vi "Write--move.vi"(8 "error in (no error)":errorcluster, 10 "Comando":T1 {"Tipo de paso" items=["Medio paso", "Paso completo"]; "Dirección" items=["Izquierda", "Derecha"]; "Tipo" items=["Unipolar", "Bipolar"]}, 11 "VISA resource name":refnum<visa-resource-name>) -> (0 "error out":errorcluster, 2 "Comando(string)":string, 3 "VISA resource name out":refnum<visa-resource-name>)   [LabVIEW 2020, in "Control de MaP.lvlib"]
doc: "Sends the move command to the MCU based in the parameters specified in the Command cluster. The MCU will be execute in a \"Moving\" state. You can send position, end-stop, all information and stop commands while in this state."
uses:
  Control de MaP.lvlib
  Controls/Command to motor.ctl
  <vilib>/Instr/_visa.llb/VISA Flush IO Buffer Mask.ctl
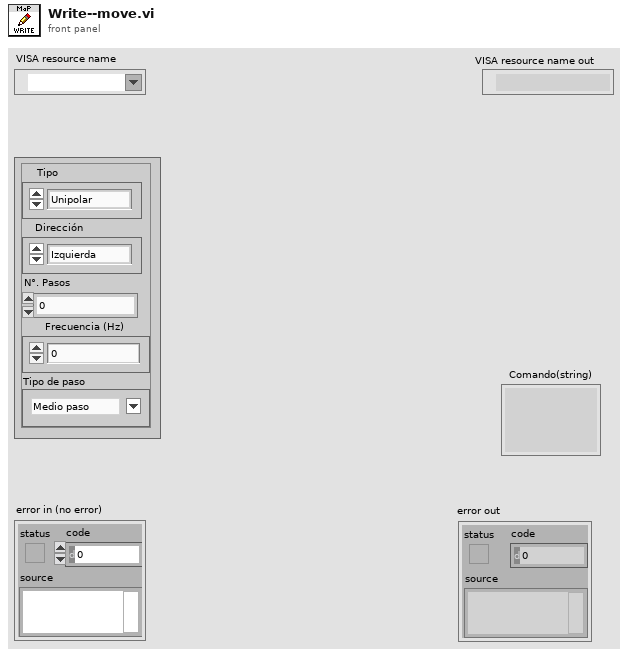
[diagram p1: front panel]
types:
  T1 = typedef "Control de MaP.lvlib/Command to motor.ctl" = cluster{"Tipo":u8, "Dirección":u8, "N°. Pasos":u16, "Frecuencia (Hz)":u8, "Tipo de paso":u8}
  T2 = typedef "VISA Flush IO Buffer Mask.ctl" = u16
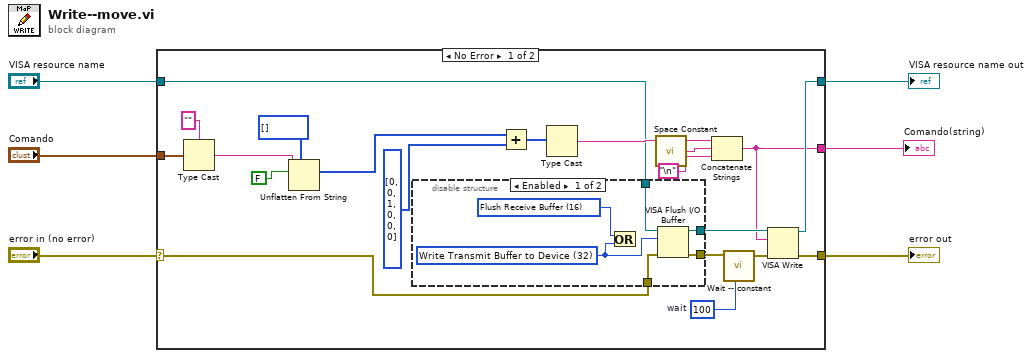
[diagram p0: block diagram]
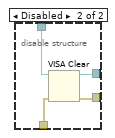
[diagram p2: hidden frame]
diagram:
  n1 = case shown="No Error" "error in (no error)" {
    selector: "error in (no error)" -> [w11 w38]
    tunnel: "VISA resource name" -> [w10 w37]
    tunnel: [w26 w37] -> w5
    tunnel: [w25 w38] -> w3
    tunnel: "Comando" -> [w24 _]
    tunnel: [w14 _] -> w1
    frame No Error {
      w9 = u32 100  # wait
      n2 = Type Cast(type="", x=w24) -> (*(type *) &x=w23:string)
      n3 = Unflatten From String(type=u8[] [], binary string=w23, data includes array or string size? (T)=FALSE) -> (value=w19:u8[])  [unwired: 2 in, 2 out]
      n4 = disable-structure shown="Enabled" {
        disable-tunnel: w11 -> [w32 w33]
        disable-tunnel: w10 -> [w31 w34]
        disable-tunnel: [w30 w35] -> w15
        disable-tunnel: [w29 w36] -> w13
        frame Enabled {
          w27 = T2 32 items=["Flush Receive Buffer"=16, "Write Transmit Buffer to Device"=32, "Flush Receive Buffer (No I/O)"=64, "Flush Transmit Buffer"=128] ("Mask")
          w28 = T2 16 items=["Flush Receive Buffer"=16, "Write Transmit Buffer to Device"=32, "Flush Receive Buffer (No I/O)"=64, "Flush Transmit Buffer"=128] ("Mask")
          n5 = Or(x=w28, y=w27) -> ()  [unwired: 1 out]
          n6 = VISA Flush I/O Buffer(VISA resource name=w31, mask (16)=w27, error in (no error)=w32) -> (VISA resource name out=w30:refnum<visa-resource-name>, error out=w29:errorcluster)
        }
        frame Disabled {
          n7 = VISA Clear(VISA resource name=w34, error in (no error)=w33) -> (VISA resource name out=w35:refnum<visa-resource-name>, error out=w36:errorcluster)
        }
      }
      n8 = Add(x=w19, y=u8[] [0, 0, 1, 0, 0, 0]) -> (x+y=w17:u8[])
      n9 = Type Cast(x=w17) -> (*(type *) &x=w16:string)  [unwired: 1 in]
      n10 = call <vilib>:"Space Constant.vi"() -> ("String"=w8:string)
      n11 = Concatenate Strings(w16, w8, "\n") -> (w14:string)
      n12 = call "Wait -- constant.vi"("error in (no error)"=w13, "wait (100 ms)"=w9) -> ("error out"=w12:errorcluster)  [unwired: 5 in]
      n13 = VISA Write(VISA resource name=w15, write buffer=w14, error in (no error)=w12) -> (VISA resource name out=w26:refnum<visa-resource-name>, error out=w25:errorcluster)  [unwired: 1 out]
    }
    frame Error {
    }
  }
  "VISA resource name out" <- w5
  "error out" <- w3
  "Comando(string)" <- w1
